vi "MDML_connect.vi"(10 "User Info":T1, 11 "client":string) -> (0 "error out":errorcluster, 1 "error out 2":errorcluster, 2 "connStatus":T2, 3 "mqtt out":refnum<class "mqtt.lvclass">, 5 "sessionPresent":bool)   [LabVIEW 2018]
uses:
  Downloads/mqtt_lv2013_201708181938/mqtt_lv2013/mqtt Folder/src/class/mqtt/mqtt.lvclass
  Downloads/mqtt_lv2013_201708181938/mqtt_lv2013/mqtt Folder/src/class/mqtt/mqttTypedef/mqttConnectionStatus.ctl
  Downloads/mqtt_lv2013_201708181938/mqtt_lv2013/mqtt Folder/src/class/mqtt/mqttTypedef/mqttWillInformation.ctl
  Downloads/mqtt_lv2013_201708181938/mqtt_lv2013/mqtt Folder/src/class/mqtt/mqttTypedef/mqttBroker.ctl
  Downloads/mqtt_lv2013_201708181938/mqtt_lv2013/mqtt Folder/src/class/mqtt/mqttTypedef/mqttConnectionFlags.ctl
  Downloads/mqtt_lv2013_201708181938/mqtt_lv2013/mqtt Folder/src/class/mqtt/mqttConfigFunction.ctl
  Downloads/mqtt_lv2013_201708181938/mqtt_lv2013/mqtt Folder/src/class/mqtt/mqttTXqueue/mqttTXdataQueueFunction.ctl
  Downloads/mqtt_lv2013_201708181938/mqtt_lv2013/mqtt Folder/src/class/mqtt/mqttTXqueue/mqttRXsubscriptionEventFunction.ctl
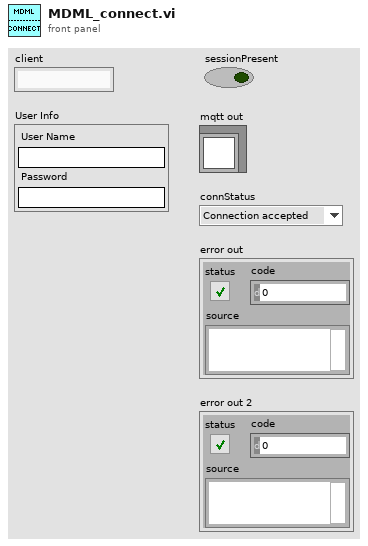
[diagram p1: front panel]
types:
  T1 = typedef "mqttWillInformation.ctl" = cluster{"User Name":string, "Password":string}
  T2 = typedef "mqttConnectionStatus.ctl" = enum16{"Connection accepted", "Connection refused: unacceptable protocol version", "Connection refused: identifier rejected", "Connection refused: Server unavailable", "Connection refused: bad user name or password", "Connection refused: not authorized"}
  T3 = typedef "mqttRXsubscriptionEventFunction.ctl" = enum16{"init", "deinit", "getEventRef", "event"}
  T4 = typedef "mqttTXdataQueueFunction.ctl" = enum16{"init", "deinit", "getQueue", "enqueue"}
  T5 = typedef "mqtt.lvclass/mqttConfigFunction.ctl" = enum16{"init", "deinit", "set", "get"}
  T6 = typedef "mqttConnectionFlags.ctl" = cluster{"reserved":bool, "clean session":bool, "will flag":bool, "willQOS":enum8{"At most once", "At least once", "Exactly once", "Reserved"}, "will retain":bool, "password":bool, "user name":bool}
  T7 = typedef "mqttBroker.ctl" = cluster{"address":string, "port":u16, "connTimeout":i32, "writeTimeout":i32, "readTimeout":i32, "subTimeout":i32}
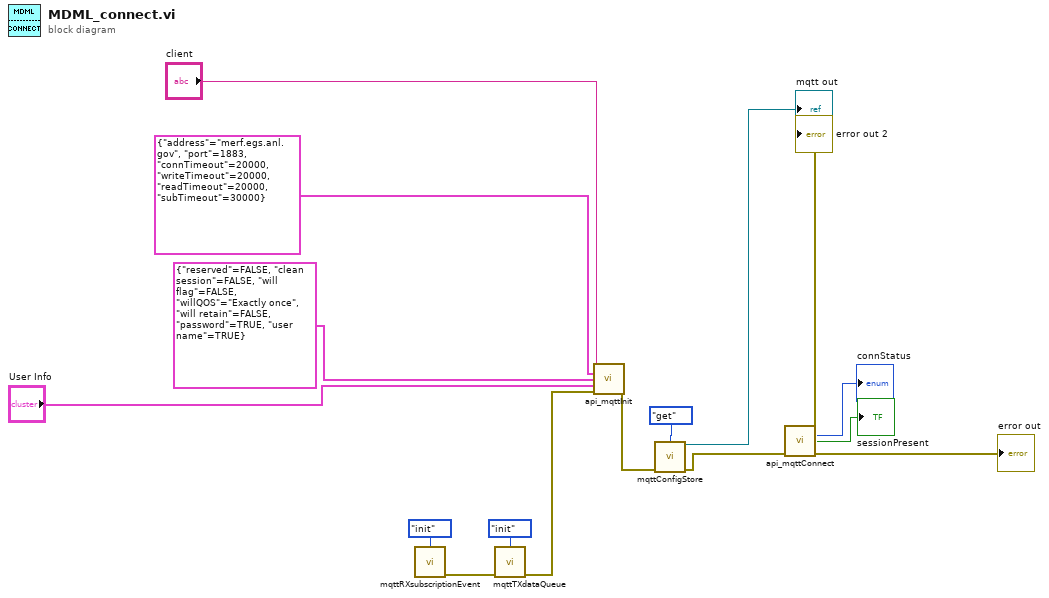
[diagram p0: block diagram]
diagram:
  n1 = call "mqttRXsubscriptionEvent.vi"("function"=mqttRXsubscriptionEventFunction."init") -> ("error out"=w11:errorcluster)  [unwired: 13 in, 1 out]
  n2 = call "mqttTXdataQueue.vi"("function"=mqttTXdataQueueFunction."init", "error in (no error)"=w11) -> ("error out"=w13:errorcluster)  [unwired: 12 in, 1 out]
  n3 = call "api_mqttInit.vi"("client"="client", "broker"=T7 {"address"="merf.egs.anl.gov", "port"=1883, "connTimeout"=20000, "writeTimeout"=20000, "readTimeout"=20000, "subTimeout"=30000}, "connFlags"=T6 {"reserved"=FALSE, "clean session"=FALSE, "will flag"=FALSE, "willQOS"=enum."Exactly once", "will retain"=FALSE, "password"=TRUE, "user name"=TRUE}, "User Info"="User Info", "error in (no error)"=w13) -> ("error out"=w7:errorcluster)  [unwired: 10 in]
  n4 = call "mqttConfigStore.vi"("function"=mqttConfigFunction."get", "error in (no error)"=w7) -> ("mqtt.lvclass out"=→"mqtt out":refnum<class "mqtt.lvclass">, "error out"=w14:errorcluster)  [unwired: 12 in]
  "error out 2" <- w14
  n5 = call "api_mqttConnect.vi"("error in (no error)"=w14) -> ("connStatus"=→"connStatus":T2, "sessionPresent"=→"sessionPresent":bool, "error out"=→"error out":errorcluster)  [unwired: 11 in, 1 out]
